vi "Log drive speed.vi"() -> ()   [LabVIEW 2013]
uses:
  Robot Global Data.vi
  <vilib>/Utility/file.llb/Write To Spreadsheet File (DBL).vi
panel:
  out "Left Rate":dbl
  out "Right Rate":dbl
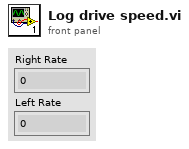
[diagram p1: front panel]
types:
  T1 = typedef "WPI_EncoderDevRef.ctl" = cluster{"DevStatus":errorcluster, "EncoderIndex":T2, "CounterIndex":T3, "DistancePerCount":dbl, "Decoding Type":T4}
  T2 = typedef "FPGA_EncoderIdx.ctl" = enum8{"Enc 0", "Enc 1", "Enc 2", "Enc 3", "Invalid"}
  T3 = typedef "FPGA_CounterCtrSystemIndex.ctl" = enum8{"Ctr 0", "Ctr 1", "Ctr 2", "Ctr 3", "Ctr 4", "Ctr 5", "Ctr 6", "Ctr 7", "Invalid"}
  T4 = typedef "WPI_EncoderType.ctl" = enum16{"1x", "2x", "4x"}
  T5 = typedef "WPI_DriverStationRobotMode2.ctl" = enum16{"Autonomous Disabled", "Autonomous Enabled", "Teleop Disabled", "Teleop Enabled", "Timeout", "Finish", "Test Disabled", "Test Enabled"}
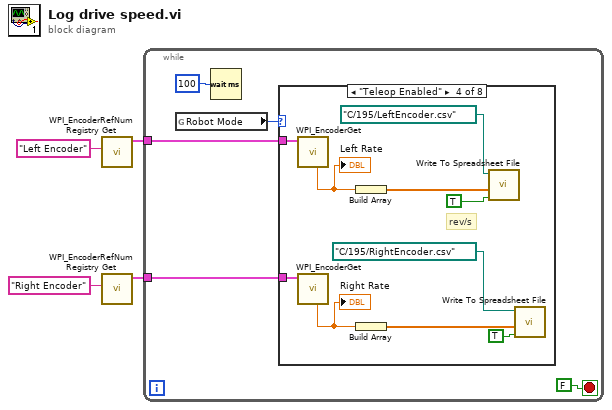
[diagram p0: block diagram]
diagram:
  n1 = call <vilib>:"WPI_EncoderRefNum Registry Get.vi"("refnum name"="Left Encoder") -> ("EncoderDevRef"=w2:T1)  [unwired: 9 in, 1 out]
  n2 = call <vilib>:"WPI_EncoderRefNum Registry Get.vi"("refnum name"="Right Encoder") -> ("EncoderDevRef"=w1:T1)  [unwired: 9 in, 1 out]
  n3 = while {
    tunnel: w2 -> [w7]
    tunnel: w1 -> [w6]
    stop <- FALSE stop-if-true
    n4 = global read "Robot Global Data.vi" "Robot Mode"() -> (w5:T5)
    n5 = Wait (ms)(milliseconds to wait=u32 100) -> ()  [unwired: 1 out]
    n6 = case shown="\"Teleop Enabled\"" w5 {
      tunnel: w7 -> [_ _ _ w15 _ _ _ _]
      tunnel: w6 -> [_ _ _ w14 _ _ _ _]
      frame "Autonomous Disabled", Default {
      }
      frame "Autonomous Enabled" {
      }
      frame "Teleop Disabled" {
      }
      frame "Teleop Enabled" {
        # "rev/s"
        n7 = call <vilib>:"WPI_EncoderGet.vi"("EncoderDevRef"=w15) -> ("Rate"=w10:dbl)  [unwired: 5 in, 5 out]
        "Left Rate" <- w10
        n8 = call <vilib>:"WPI_EncoderGet.vi"("EncoderDevRef"=w14) -> ("Rate"=w12:dbl)  [unwired: 5 in, 5 out]
        "Right Rate" <- w12
        n9 = Build Array(w10) -> (w13:dbl[])
        n10 = Build Array(w12) -> (w11:dbl[])
        n11 = call-poly <vilib>:"Write To Spreadsheet File.vi"("append to file? (new file:F)"=TRUE, "1D data"=w13, "file path (dialog if empty)"=path "C:/195/LeftEncoder.csv") -> ()  [unwired: 5 in, 1 out]
        n12 = call-poly <vilib>:"Write To Spreadsheet File.vi"("append to file? (new file:F)"=TRUE, "1D data"=w11, "file path (dialog if empty)"=path "C:/195/RightEncoder.csv") -> ()  [unwired: 5 in, 1 out]
      }
      frame "Timeout" {
      }
      frame "Finish" {
      }
      frame "Test Disabled" {
      }
      frame "Test Enabled" {
      }
    }
  }
